vi "update.startTime.request.vi"(8 "error in":errorcluster, 10 "Start Time (empty: now)":timestamp format="%<%x %.3X>T", 11 "event":refnum<class "event.lvclass">) -> (0 "error out":errorcluster, 3 "request":string)   [LabVIEW 2020, in "event.lvclass"]
uses:
  event.lvclass
  event.lvclass/event.ctl
  7f973197-732c-47a5-8c43-195cf15d244e.vi
  <vilib>/LabVIEW Open Source Project/Epoch Date & Time/epoch.UNIX/Epoch.UNIX.lvclass
  C:/Program Files/National Instruments/LabVIEW 2020/vi.lib/LabVIEW Open Source Project/Epoch Date & Time/epoch/Epoch.lvclass
  <vilib>/LabVIEW Open Source Project/Epoch Date & Time/Get Epoch Time.vi
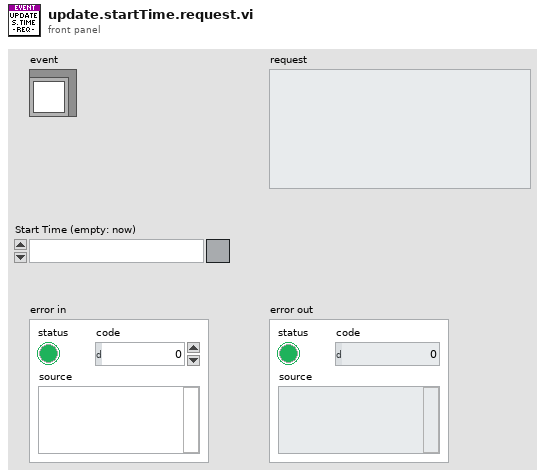
[diagram p1: front panel]
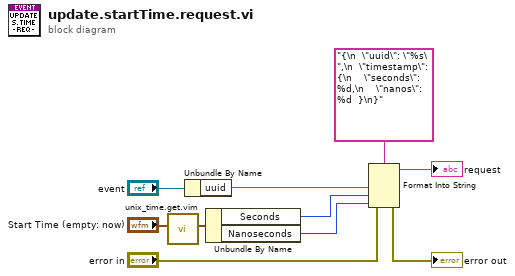
[diagram p0: block diagram]
diagram:
  n1 = call "unix_time.get.vim"("Time Stamp (empty: now) [single or array]"="Start Time (empty: now)") -> ("UNIX Timestamp"=w4:cluster{"Seconds":i64, "Nanoseconds":i64})  [unwired: 10 in]
  n2 = Unbundle By Name("event") -> ("uuid"=w8:string)
  n3 = Unbundle By Name(w4) -> ("Seconds"=w2:i64, "Nanoseconds"=w1:i64)
  n4 = Format Into String(format string="{\n  \"uuid\": \"%s\",\n  \"timestamp\": {\n    \"seconds\": %d,\n    \"nanos\": %d  }\n}", error in="error in", w8, w2, w1) -> (resulting string=→"request":string, error out=→"error out":errorcluster)  [unwired: 1 in]
